vi "Write Configuration File.vi"(8 "error in (no error)":errorcluster, 11 "Example Instrument in":refnum<class "Instrument.Template.lvclass">) -> (0 "error out":errorcluster, 3 "Example Instrument out":refnum<class "Instrument.Template.lvclass">)   [LabVIEW 2019, in "Instrument.Template.lvclass"]
uses:
  Instrument.Template.lvclass
  C:/Users/patrick/Documents/GitHub/Instrument-Framework/lvsrc/SMOs/Instrument/Instrument.lvclass
  SMOs/Instrument/Instrument.lvclass/Instrument.ctl
  Instrument.Template.lvclass/Instrument.Template.ctl
  SMOs/Configuration/Configuration.lvclass
  SMOs/Instrument/Instrument.lvclass
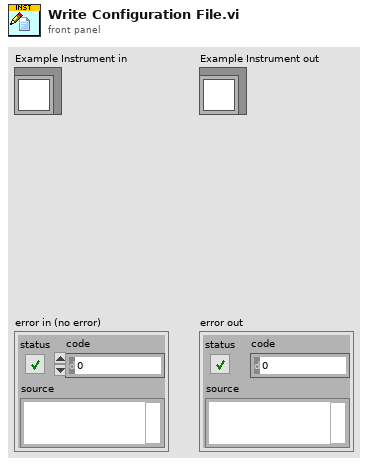
[diagram p1: front panel]
types:
  T1 = typedef "Instrument.Template.lvclass/Instrument.Template.Configuration--Cluster.ctl" = cluster{"Example Setting 1":dbl, "Example Setting 2":dbl, "Example Setting 3":string}
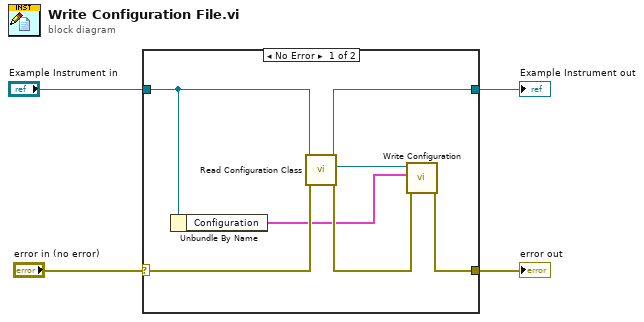
[diagram p0: block diagram]
diagram:
  n1 = case shown="No Error" "error in (no error)" {
    selector: "error in (no error)" -> [w7 w13]
    tunnel: "Example Instrument in" -> [w6 w12]
    tunnel: [w10 w12] -> w3
    tunnel: [w9 w13] -> w2
    frame No Error {
      n2 = Unbundle By Name(w6) -> ("Configuration"=w5:T1)
      n3 = call "Read Configuration Class.vi"("error in (no error)"=w7, "Instrument in"=w6) -> ("error out"=w11:errorcluster, "Configuration.lvclass"=w8:refnum<class "Configuration.lvclass">, "Instrument out"=w10:refnum<class "Instrument.Template.lvclass">)  [unwired: 7 in]
      n4 = call "Write Configuration.vi"("error in (no error)"=w11, "Variant"=w5, "Configuration in"=w8) -> ("error out"=w9:errorcluster)  [unwired: 7 in, 1 out]
    }
    frame Error {
    }
  }
  "Example Instrument out" <- w3
  "error out" <- w2
